vi "Configure Mode.vi"(8 "error in (no error)":errorcluster, 10 "mode":T1, 11 "TroSpec in":refnum<class "PL ISTEQ TroSpec.lvclass">) -> (0 "error out":errorcluster, 3 "TroSpec out":refnum<class "PL ISTEQ TroSpec.lvclass">)   [LabVIEW 2015, in "PL ISTEQ TroSpec.lvclass"]
doc: "Configures CCD mode."
uses:
  PL ISTEQ TroSpec.lvclass
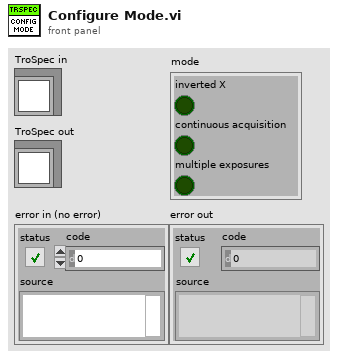
[diagram p1: front panel]
types:
  T1 = cluster{"inverted X":bool, "continuous acquisition":bool, "multiple exposures":bool}
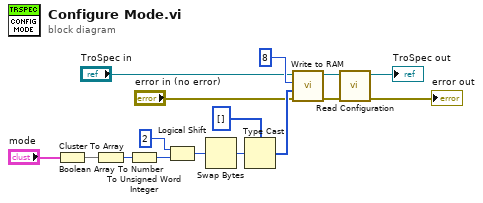
[diagram p0: block diagram]
diagram:
  n1 = Cluster To Array(cluster="mode") -> (array=w9:bool[])
  n2 = Boolean Array To Number(Boolean array=w9) -> (number=w8:u32)
  n3 = To Unsigned Word Integer(number=w8) -> (unsigned 16bit integer=w7:u16)
  n4 = Logical Shift(y=i16 2, x=w7) -> (x << y=w5:u16)
  n5 = Swap Bytes(anything=w5) -> (byte swapped=w11:u16)
  n6 = Type Cast(type=u8[] [] ("data"), x=w11) -> (*(type *) &x=w16:u8[])
  n7 = call "Write to RAM.vi"("error in (no error)"="error in (no error)", "data"=w16, "address"=u16 8, "TroSpec in"="TroSpec in") -> ("error out"=w3:errorcluster, "TroSpec out"=w4:refnum<class "PL ISTEQ TroSpec.lvclass">)  [unwired: 6 in]
  n8 = call "Read Configuration.vi"("error in (no error)"=w3, "TroSpec in"=w4) -> ("error out"=→"error out":errorcluster, "TroSpec out"=→"TroSpec out":refnum<class "PL ISTEQ TroSpec.lvclass">)  [unwired: 7 in, 1 out]
